vi "Feedback-node-sample.vi"() -> ()   [LabVIEW 2020]
panel:
  out "Previous\nValue":i32
  in  "stop\nloop":bool
  out "Loop\nCount":i32
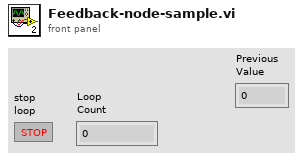
[diagram p1: front panel]
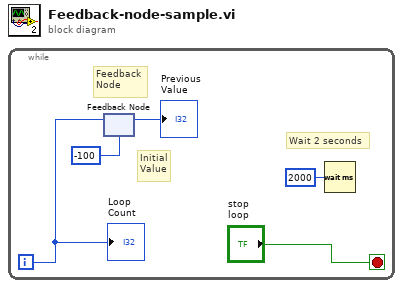
[diagram p0: block diagram]
diagram:
  n1 = while {
    i -> [w3]
    stop <- "stop\nloop" stop-if-true
    # "Feedback\nNode"
    # "Initial\nValue"
    # "Wait 2 seconds"
    n2 = feedback-in #1(w3) -> ()
    n3 = feedback #1(-100) -> (→"Previous\nValue":i32)
    n4 = Wait (ms)(milliseconds to wait=u32 2000) -> ()  [unwired: 1 out]
    "Loop\nCount" <- w3
  }
